vi "GetColor.vi"(8 "error in (no error)":errorcluster, 11 "ColorRGB in":refnum<class "ColorRGB.lvclass">) -> (0 "error out":errorcluster, 2 "Color":u32(colorbox), 3 "ColorRGB out":refnum<class "ColorRGB.lvclass">)   [LabVIEW 2021, in "Picture2D.lvlib" / "ColorRGB.lvclass"]
uses:
  ColorRGB.lvclass
  Color/Color.lvclass
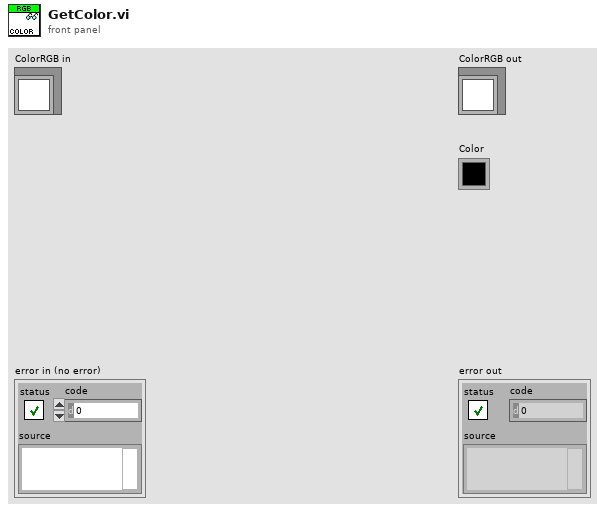
[diagram p1: front panel]
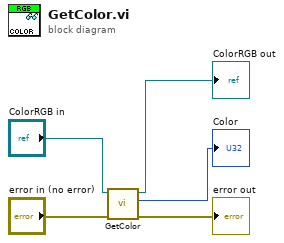
[diagram p0: block diagram]
diagram:
  n1 = call-parent "GetColor.vi"("error in (no error)"="error in (no error)", "Color in"="ColorRGB in") -> ("error out"=→"error out":errorcluster, "Color"=→"Color":u32, "Color out"=→"ColorRGB out":refnum<class "ColorRGB.lvclass">)  [unwired: 7 in]
